vi "Set Cell Color and Border.vi"(1 "Border edges":T2={"Left   "=TRUE, "Right"=TRUE, "Top"=TRUE, "Bottom"=TRUE, "All"=FALSE}, 2 "Border style":T1, 4 "Fill Color":u32(colorbox), 5 "Border Color":u32(colorbox), 6 "Apply Fill":bool, 7 "Apply Border":bool, 8 "error in (no error)":errorcluster, 9 "End Cell Address":string, 10 "Start Cell Address":string, 11 "Report Ref In":T3) -> (0 "error out":errorcluster, 3 "Report Ref Out":T3)   [LabVIEW 2013, in "XCel Report Engine.lvlib"]
doc: "Applies background fill and border formatting to a cell or rectangular cell range in the active worksheet.\n\nStart Cell Address and End Cell Address use Excel A1 notation. If End Cell Address is empty, formatting is applied only to Start Cell Address.\n\nWhen Apply Fill is TRUE, Fill Color is applied as a solid cell background. When Apply Border is TRUE, Border Color and Border Style are applied to the edges selected by Border Edges.\n\nFill and border formatting can be enabled independently. A formatting category that is not enabled remains unchanged.\n\nWhen applied to a range, the selected borders are formatted on every individual cell in the range. Selecting all four edges therefore produces a cell grid, not only an outer border around the complete range.\n\nThe operation preserves cell values, formulas, and unrelated formatting properties.\n\nAn error is returned if either cell address is invalid, the end cell precedes the start cell, or a formatting value is unsupported."
uses:
  XCel Report Engine.lvlib
  C:/Users/m.santucci/Documents/ChatGPT/LV_REPORT_ENGINE/LV/DotNet/XCelReportEngine.dll
  LV/DotNet/XCelReportEngine.dll
  Controls/Report Ref.ctl
  Controls/Border edges.ctl
  Controls/Border style.ctl
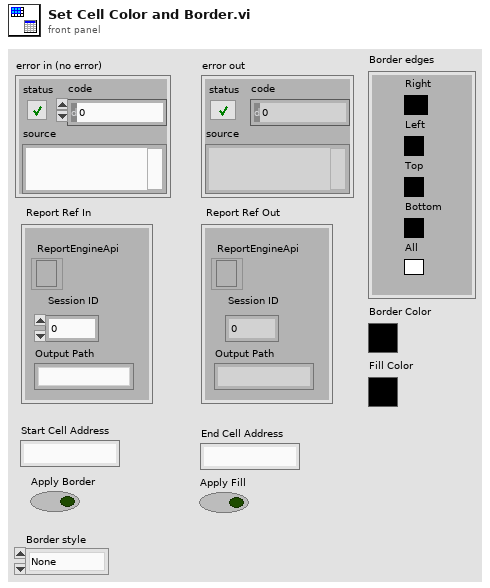
[diagram p1: front panel]
types:
  T1 = typedef "XCel Report Engine.lvlib/Border style.ctl" = enum16{"None", "Thin", "Medium", "Thick", "Double", "Dashed", "Dotted"}
  T2 = typedef "XCel Report Engine.lvlib/Border edges.ctl" = cluster{"Left   ":bool, "Right":bool, "Top":bool, "Bottom":bool, "All":bool}
  T3 = typedef "XCel Report Engine.lvlib/Report Ref.ctl" = cluster{"Session ID":i32, "Output Path":string, "ReportEngineApi":refnum<k24>}
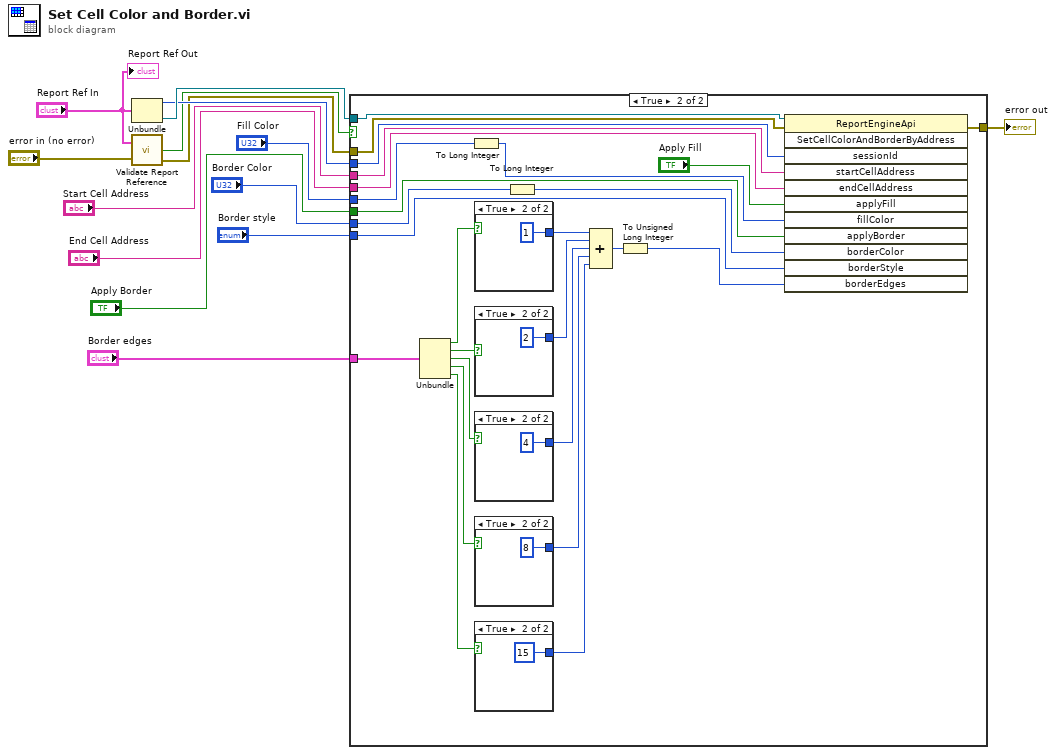
[diagram p0: block diagram]
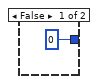
[diagram p3: hidden frame]
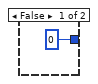
[diagram p4: hidden frame]
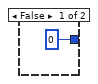
[diagram p5: hidden frame]
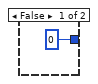
[diagram p6: hidden frame]
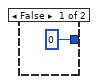
[diagram p7: hidden frame]
diagram:
  n1 = Unbundle("Report Ref In") -> ("Session ID"=w12:i32, "ReportEngineApi"=w14:refnum<k24>)  [unwired: 1 out]
  n2 = call "Validate Report Reference.vi"("Report Ref In"="Report Ref In", "error in (no error)"="error in (no error)") -> ("Valid"=w7:bool, "error out"=w8:errorcluster)  [unwired: 1 out]
  n3 = case shown="True" w7 {
    tunnel: w14 -> [_ w41]
    tunnel: [w15 w40] -> w13
    tunnel: w12 -> [_ w39]
    tunnel: "Border edges" -> [_ w37]
    tunnel: w8 -> [w15 w22]
    tunnel: "Fill Color" -> [_ w21]
    tunnel: "Border Color" -> [_ w20]
    tunnel: "Apply Border" -> [_ w19]
    tunnel: "End Cell Address" -> [_ w18]
    tunnel: "Start Cell Address" -> [_ w17]
    tunnel: "Border style" -> [_ w16]
    frame False {
    }
    frame True {
      n4 = Unbundle(w37) -> ("Left"=w36:bool, "Right"=w35:bool, "Top"=w34:bool, "Bottom"=w33:bool, "All"=w32:bool)
      n5 = To Long Integer(number=w21) -> (32bit integer=w23:i32)
      n6 = case shown="True" w36 {
        tunnel: [0 1] -> w31
        frame False {
        }
        frame True {
        }
      }
      n7 = case shown="True" w35 {
        tunnel: [0 2] -> w30
        frame False {
        }
        frame True {
        }
      }
      n8 = case shown="True" w34 {
        tunnel: [0 4] -> w29
        frame False {
        }
        frame True {
        }
      }
      n9 = case shown="True" w33 {
        tunnel: [0 8] -> w28
        frame False {
        }
        frame True {
        }
      }
      n10 = case shown="True" w32 {
        tunnel: [0 15] -> w27
        frame False {
        }
        frame True {
        }
      }
      n11 = To Long Integer(number=w20) -> (32bit integer=w24:i32)
      n12 = Compound Arithmetic op=ADD(w31, w30, w29, w28, w27) -> (w26:i32)
      n13 = To Unsigned Long Integer(number=w26) -> (unsigned 32bit integer=w25:u32)
      n14 = invoke class="ReportEngineApi" method="SetCellColorAndBorderByAddress"(reference=w41, error in=w22, "sessionId"=w39, "startCellAddress"=w17, "endCellAddress"=w18, "applyFill"="Apply Fill", "fillColor"=w23, "applyBorder"=w19, "borderColor"=w24, "borderStyle"=w16, "borderEdges"=w25) -> (error out=w40:errorcluster)  [unwired: 1 in, 11 out]
    }
  }
  "error out" <- w13
  "Report Ref Out" <- "Report Ref In"
